vi "FPGA_SystemFPGA Ref Global.vi"() -> ()   [LabVIEW 2018]
panel:
  out "FRC FPGA Status":errorcluster
  out "FRC FPGA Ref":refnum<k20>
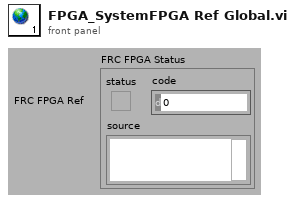
[diagram p1: front panel]
diagram:
